vi "GV_Lock State.vi"() -> ()   [LabVIEW 2015]
panel:
  in  "GV_Lock State":dbl
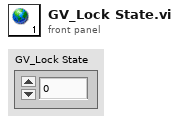
[diagram p1: front panel]
diagram:
